vi "Test Find Edges.vi"(11 "Camera Image":T1(plugin-control)=refnum) -> ()   [LabVIEW 2025]
uses:
  <vilib>/vision/NI_Vision_Development_Module.lvlib
panel:
  out "size(s)":i32[](array[numeric])
  in  "Max Score":dbl
  in  "Min Score":dbl
  in  "Threshold":dbl=500.0 format="%#_13g"
  out "Extracted Image":T1(plugin-control)
  out "Score":dbl[](array[numeric])
  out "Particle Measurements (Pixels) 2":dbl[][](array[numeric])
  out "Particle Measurements (Pixels)":dbl[][](array[numeric]) format="%.2f"
  out "Number of Particles":i32
  out "Treshold":T1(plugin-control)
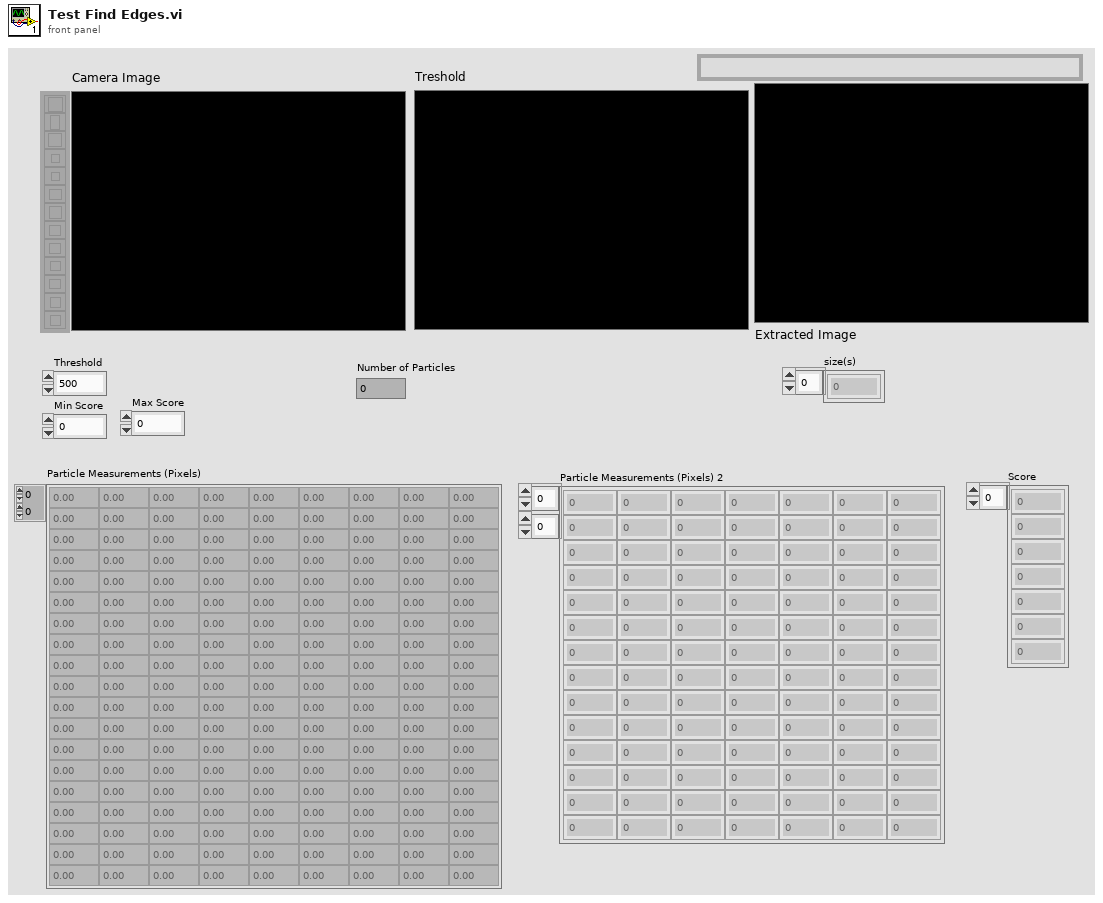
[diagram p1: front panel]
types:
  T1 = typedef "IMAQ Image.ctl" = refnum<image>
  T2 = typedef "Particle Parameters" = i32
  T3 = typedef "Image Type" = u32
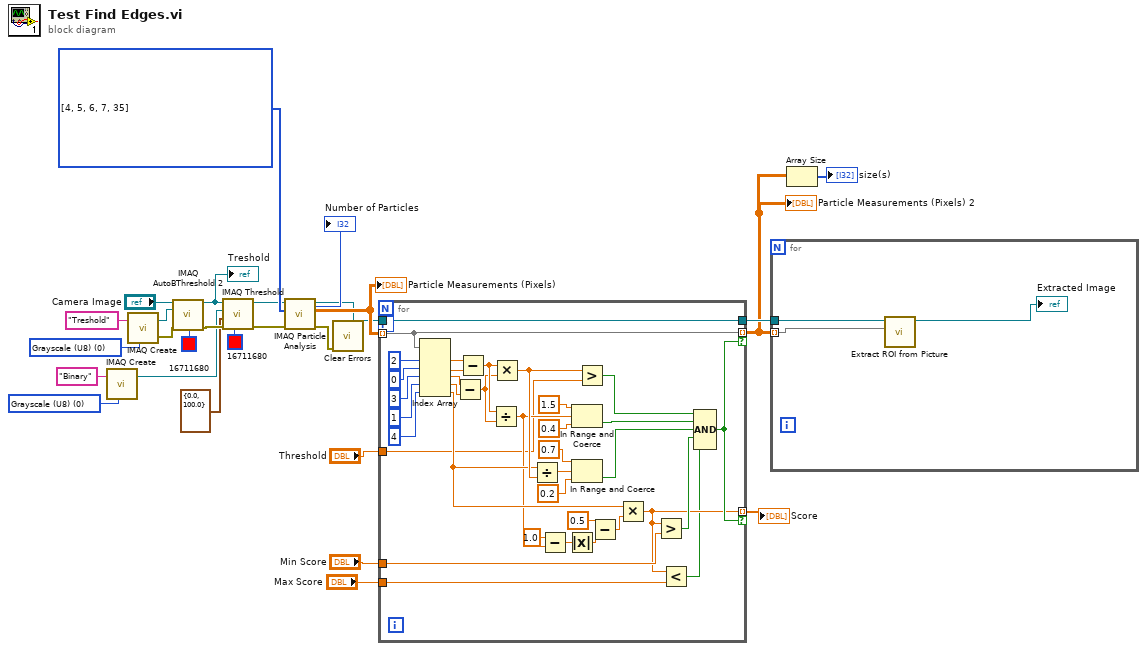
[diagram p0: block diagram]
diagram:
  w13 = T2[] [4, 5, 6, 7, 35] items=["Center of Mass X", "Center of Mass Y", "First Pixel X", "First Pixel Y", "Bounding Rect Left", "Bounding Rect Top", "Bounding Rect Right", "Bounding Rect Bottom", "Max Feret Diameter Start X", "Max Feret Diameter Start Y", "Max Feret Diameter End X", "Max Feret Diameter End Y", "Max Horiz. Segment Length Left", "Max Horiz. Segment Length Right", "Max Horiz. Segment Length Row", "-", "Bounding Rect Width", "Bounding Rect Height", "Bounding Rect Diagonal", "Perimeter", "Convex Hull Perimeter", "Holes' Perimeter", "Max Feret Diameter", "Equivalent Ellipse Major Axis", "Equivalent Ellipse Minor Axis", "Equivalent Ellipse Minor Axis (Feret)", "Equivalent Rect Long Side", "Equivalent Rect Short Side", "Equivalent Rect Diagonal", "Equivalent Rect Short Side (Feret)", "Average Horiz. Segment Length", "Average Vert. Segment Length", "Hydraulic Radius", "Waddel Disk Diameter", "-", "Area", "Holes' Area", "Particle & Holes' Area", "Convex Hull Area", "Image Area", "-", "Number of Holes", "Number of Horiz. Segments", "Number of Vert. Segments", "-", "Orientation", "Max Feret Diameter Orientation", "-", "% Area/Image Area", "% Area/(Particle & Holes' Area)", "Ratio of Equivalent Ellipse Axes", "Ratio of Equivalent Rect Sides", "-", "Elongation Factor", "Compactness Factor", "Heywood Circularity Factor", "Type Factor", "-", "Sum X", "Sum Y", "Sum XX", "Sum XY", "Sum YY", "Sum XXX", "Sum XXY", "Sum XYY", "Sum YYY", "-", "Moment of Inertia XX", "Moment of Inertia XY", "Moment of Inertia YY", "Moment of Inertia XXX", "Moment of Inertia XXY", "Moment of Inertia XYY", "Moment of Inertia YYY", "Norm. Moment of Inertia XX", "Norm. Moment of Inertia XY", "Norm. Moment of Inertia YY", "Norm. Moment of Inertia XXX", "Norm. Moment of Inertia XXY", "Norm. Moment of Inertia XYY", "Norm. Moment of Inertia YYY", "Hu Moment 1", "Hu Moment 2", "Hu Moment 3", "Hu Moment 4", "Hu Moment 5", "Hu Moment 6", "Hu Moment 7"] ("Pixel Measurements")
  w18 = T3 0 items=["Grayscale (U8)", "Grayscale (I16)", "Grayscale (SGL)", "Complex (CSG)", "RGB (U32)", "HSL (U32)", "RGB (U64)", "Grayscale (U16)"] ("Image Type")
  w27 = T3 0 items=["Grayscale (U8)", "Grayscale (I16)", "Grayscale (SGL)", "Complex (CSG)", "RGB (U32)", "HSL (U32)", "RGB (U64)", "Grayscale (U16)"] ("Image Type")
  n1 = call "IMAQ Create"("Image Name"="Binary", "Image Type"=w18) -> ("New Image"=w17:T1)  [unwired: 2 in, 2 out]
  n2 = call "IMAQ Create"("Image Name"="Treshold", "Image Type"=w27) -> ("New Image"=w24:T1, "error out"=w22:errorcluster)  [unwired: 2 in, 1 out]
  n3 = call "IMAQ AutoBThreshold 2"("Image Src"="Camera Image", "Image Dst"=w24, "error in (no error)"=w22, "Replace Value (1)"=u32 16711680) -> ("Image Dst Out"=w20:T1, "error out"=w19:errorcluster)  [unwired: 9 in, 1 out]
  "Treshold" <- w20
  n4 = call "IMAQ Threshold"("Replace Value"=u32 16711680, "error in (no error)"=w19, "Range"=cluster{"Lower value":sgl, "Upper value":sgl} {"Lower value"=0.0, "Upper value"=100.0}, "Image Dst"=w17, "Image Src"=w20) -> ("error out"=w8:errorcluster, "Image Dst Out"=w7:T1)  [unwired: 5 in]
  n5 = call "IMAQ Particle Analysis"("error in (no error)"=w8, "Pixel Measurements"=w13, "Image"=w7) -> ("error out"=w14:errorcluster, "Particle Measurements (Pixels)"=w12:dbl[][], "Image Out (duplicate)"=w6:T1, "Number of Particles"=→"Number of Particles":i32)  [unwired: 3 in, 2 out]
  "Particle Measurements (Pixels)" <- w12
  n6 = call <vilib>:"Clear Errors.vi"("error in (no error)"=w14) -> ()  [unwired: 5 in, 2 out]
  n7 = for {
    tunnel: w12 -> [w32] mode=indexing
    tunnel: [w32] -> w2 mode=indexing if=w37
    tunnel: [w30] -> w11 mode=indexing if=w37
    tunnel: "Threshold" -> [w35]
    tunnel: "Min Score" -> [w34]
    tunnel: w6 -> [w31]
    tunnel: [w31] -> w5
    workers-P: _ -> [_]
    tunnel: "Max Score" -> [w29]
    n8 = Index Array(array=w32, index #1=2 ("index"), index #2=0 ("index"), index #3=3 ("index"), index #4=1 ("index"), index #5=4 ("index")) -> (element #1=w58:dbl, element #2=w59:dbl, element #3=w57:dbl, element #4=w56:dbl, element #5=w43:dbl)
    n9 = Subtract(x=w57, y=w56) -> (x-y=w54:dbl)
    n10 = Subtract(x=w58, y=w59) -> (x-y=w55:dbl)
    n11 = Divide(x=w55, y=w54) -> (x/y=w41:dbl)
    n12 = Multiply(x=w55, y=w54) -> (x*y=w48:dbl)
    n13 = Divide(x=w43, y=w48) -> (x/y=w47:dbl)
    n14 = Subtract(x=1.0, y=w41) -> (x-y=w40:dbl)
    n15 = Absolute Value(x=w40) -> (abs(x)=w39:dbl)
    n16 = In Range and Coerce(upper limit=1.5, x=w41, lower limit=0.4 ("upper limit")) -> (In Range?=w50:bool)  [unwired: 1 out]
    n17 = In Range and Coerce(upper limit=0.7, x=w47, lower limit=0.2 ("upper limit")) -> (In Range?=w44:bool)  [unwired: 1 out]
    n18 = Greater?(x=w48, y=w35) -> (0:w51:bool)
    n19 = Subtract(x=0.5, y=w39) -> (x-y=w38:dbl)
    n20 = Multiply(x=w43, y=w38) -> (x*y=w30:dbl)
    n21 = Greater?(x=w30, y=w34) -> (0:w33:bool)
    n22 = Less?(x=w30, y=w29) -> (x < y?=w28:bool)
    n23 = Compound Arithmetic op=AND(w51, w50, w44, w33, w28) -> (w37:bool)
  }
  "Score" <- w11
  "Particle Measurements (Pixels) 2" <- w2
  n24 = for {
    tunnel: w2 -> [w64] mode=indexing
    tunnel: w5 -> [w66]
    n25 = call "Extract ROI from Picture.vi"("Particle Measurements (Pixels)"=w64, "Refnum in"=w66) -> ("Extracted Image"=→"Extracted Image":T1)  [unwired: 9 in]
  }
  n26 = Array Size(array=w2) -> (size(s)=→"size(s)":i32[])
